vi "MM Multi DOF State Machine.vi"(10 "Force Control Parameters":T2, 11 "Convergence Status In":T1[](array[typedef])) -> (3 "Convergence Status Out":T1[](array[typedef]))   [LabVIEW 2009]
uses:
  Data Access Objects/Mixed Mode/Force Control Parameters.ctl
  Mixed Mode Convergence Status.ctl
  Data Access Objects/Metadata/DAO Actions.ctl
  Mixed Mode Multidof State.ctl
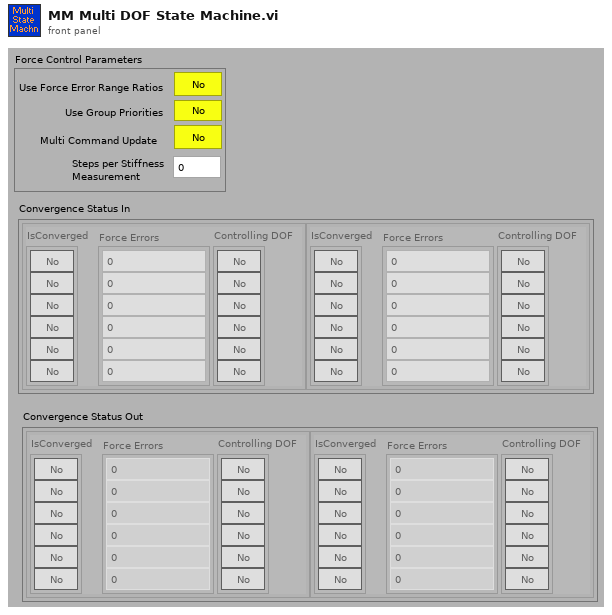
[diagram p1: front panel]
types:
  T1 = typedef "Mixed Mode Convergence Status.ctl" = cluster{"IsConverged":bool[], "Force Errors":dbl[], "Controlling DOF":bool[]}
  T2 = typedef "Force Control Parameters.ctl" = cluster{"Use Force Error Range Ratios":bool, "Use Group Priorities":bool, "Multi Command Update":bool, "Steps per Stiffness \nMeasurement":i32}
  T3 = typedef "DAO Actions.ctl" = enum16{"Init", "Get", "Set"}
  T4 = typedef "Mixed Mode Multidof Status.ctl" = cluster{"Mixed Mode Multidof State":T5, "Multi DOF Ramp Count":i32, "Stiffness Tested":T6[][]}
  T5 = typedef "Mixed Mode Multidof State.ctl" = enum16{"Multidof", "Stiffness Test"}
  T6 = typedef "Yes No Button.ctl" = bool
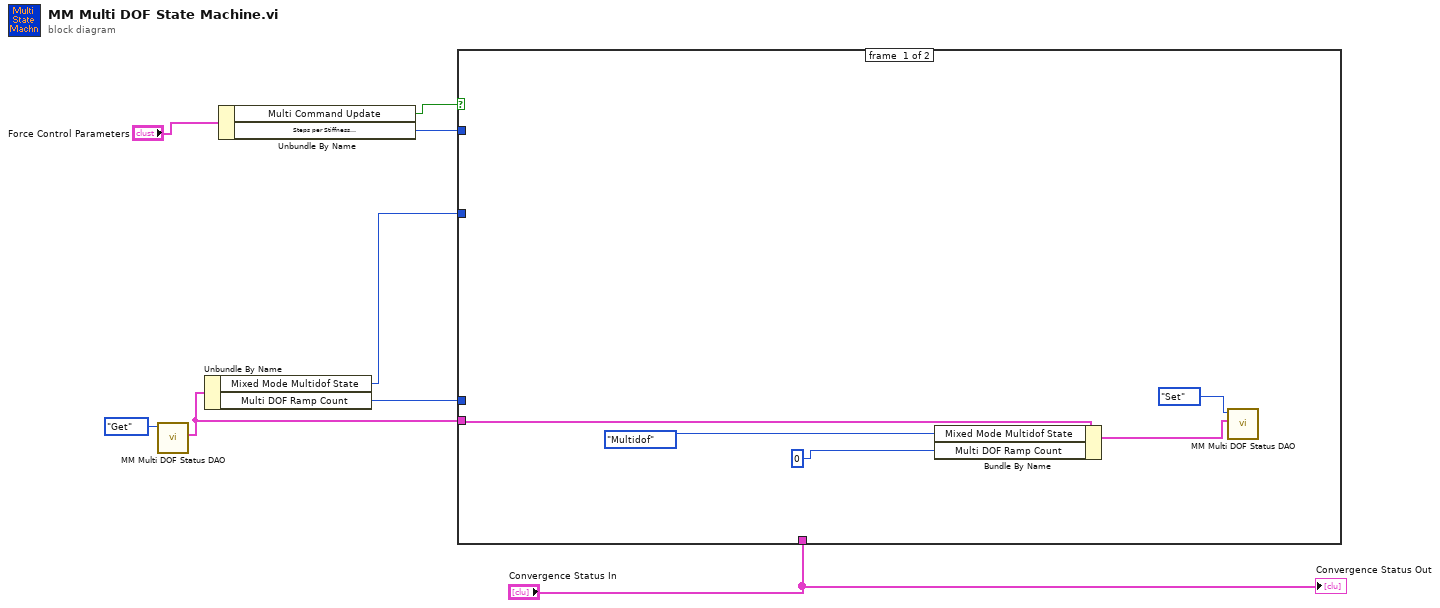
[diagram p0: block diagram]
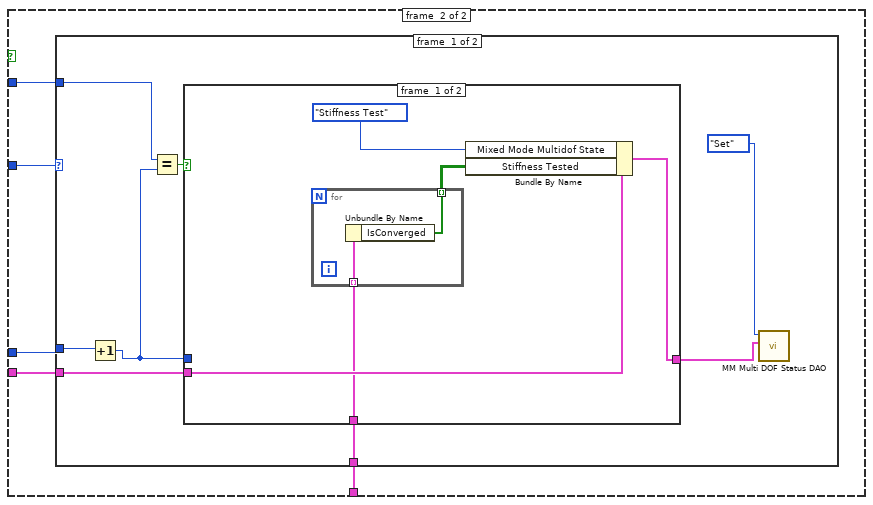
[diagram p2: hidden frame]
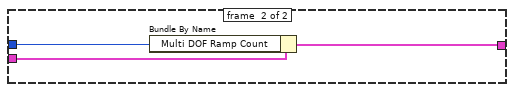
[diagram p3: hidden frame]
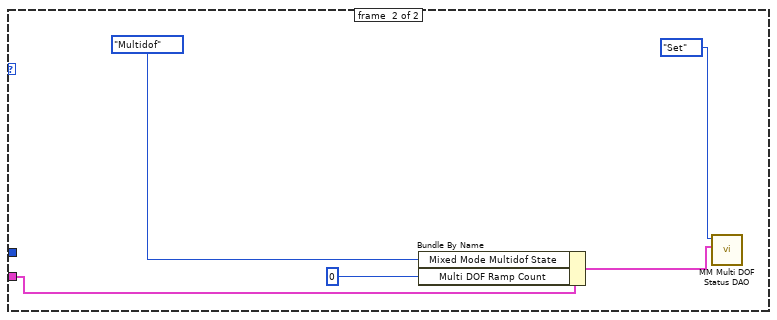
[diagram p4: hidden frame]
diagram:
  n1 = call "MM Multi DOF Status DAO.vi"("Actions"=DAO_Actions."Get") -> ("Mixed Mode Multidof Status Out"=w5:T4)  [unwired: 9 in, 1 out]
  n2 = Unbundle By Name(w5) -> ("Mixed Mode Multidof State"=w7:T5, "Multi DOF Ramp Count"=w6:i32)
  n3 = Unbundle By Name("Force Control Parameters") -> ("Multi Command Update"=w2:bool, "Steps per Stiffness \nMeasurement"=w3:i32)
  n4 = case shown="True" w2 {
    tunnel: w7 -> [_ w18]
    tunnel: w6 -> [_ w17]
    tunnel: w5 -> [w9 w16]
    tunnel: w3 -> [_ w15]
    tunnel: "Convergence Status In" -> [_ w14]
    frame #0 {
      n5 = Bundle By Name(cluster=w9, "Mixed Mode Multidof State"=Mixed_Mode_Multidof_State."Multidof", "Multi DOF Ramp Count"=0 ("Next Stiffness DOF L1")) -> (w12:T4)
      n6 = call "MM Multi DOF Status DAO.vi"("Mixed Mode Multidof Status In"=w12, "Actions"=DAO_Actions."Set") -> ()  [unwired: 8 in, 2 out]
    }
    frame #1 {
      n7 = case shown="\"Multidof\"" w18 {
        tunnel: w17 -> [w23 _]
        tunnel: w16 -> [w24 w39]
        tunnel: w15 -> [w20 _]
        tunnel: w14 -> [w19 _]
        frame #0 {
          n8 = Increment(x=w23) -> (x+1=w21:i32)
          n9 = Equal?(x=w20, y=w21) -> (x = y?=w22:bool)
          n10 = case shown="True" w22 {
            tunnel: [w31 w36] -> w25
            tunnel: w24 -> [w30 w35]
            tunnel: w21 -> [_ w34]
            tunnel: w19 -> [w28 _]
            frame #0 {
              n11 = for {
                tunnel: w28 -> [w33] mode=indexing
                tunnel: [w32] -> w27 mode=indexing
                n12 = Unbundle By Name(w33) -> ("IsConverged"=w32:bool[])
              }
              n13 = Bundle By Name(cluster=w30, "Mixed Mode Multidof State"=Mixed_Mode_Multidof_State."Stiffness Test", "Stiffness Tested"=w27) -> (w31:T4)
            }
            frame #1 {
              n14 = Bundle By Name(cluster=w35, "Multi DOF Ramp Count"=w34) -> (w36:T4)
            }
          }
          n15 = call "MM Multi DOF Status DAO.vi"("Mixed Mode Multidof Status In"=w25, "Actions"=DAO_Actions."Set") -> ()  [unwired: 8 in, 2 out]
        }
        frame #1 {
          n16 = Bundle By Name(cluster=w39, "Mixed Mode Multidof State"=Mixed_Mode_Multidof_State."Multidof", "Multi DOF Ramp Count"=0) -> (w40:T4)
          n17 = call "MM Multi DOF Status DAO.vi"("Mixed Mode Multidof Status In"=w40, "Actions"=DAO_Actions."Set") -> ()  [unwired: 8 in, 2 out]
        }
      }
    }
  }
  "Convergence Status Out" <- "Convergence Status In"
